vi "Write Application Style Reference.vi"(10 "Application Style Reference":T1, 11 "IViewable in":refnum<class "IViewable.lvclass">) -> (3 "IViewable out":refnum<class "IViewable.lvclass">)   [LabVIEW 2017, in "IViewable.lvlib" / "IViewable.lvclass"]
uses:
  IViewable.lvclass
  ApplicationStyleReference/Application Style Reference.ctl
  ApplicationStyleReference/ApplicationStyleReference.lvclass
  IViewable.lvclass/IViewable.ctl
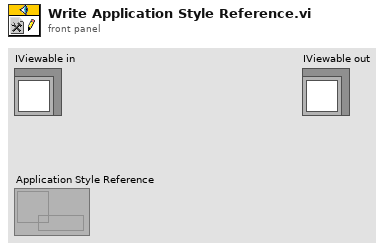
[diagram p1: front panel]
types:
  T1 = typedef "IViewable.lvlib/ApplicationStyleReference.lvclass/Application Style Reference.ctl" = refnum<data-value>
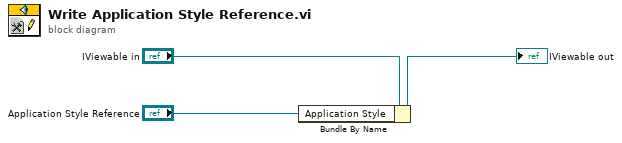
[diagram p0: block diagram]
diagram:
  n1 = Bundle By Name(cluster="IViewable in", "Application Style"="Application Style Reference") -> (→"IViewable out":refnum<class "IViewable.lvclass">)
